vi "Monta comando comFilas .vi"(6 "Set Point":string, 7 "Comando":string, 8 "Dispositivo":string, 9 "Controlador":u16(ring)=1 items=["ZERO", "AH", "DEC", "TUBO", "CUP"]) -> (0 "Erro Comunicação":bool, 1 "String Enviado":string, 2 "Resposta":string, 3 "Erro Resp":bool)   [LabVIEW 2018]
uses:
  Global_Telescopio.vi
panel:
  out "ERRO":bool
  # "PROG"
  # "SIDERAL"
  # "EMBREAGEM"
  # "DESLIGAR"
  # "STATUS"
  # "LIGAR"
  # "PARAR"
  # "ERROS"
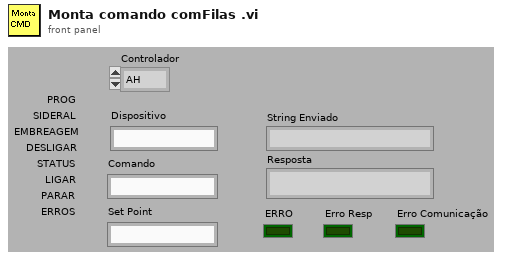
[diagram p1: front panel]
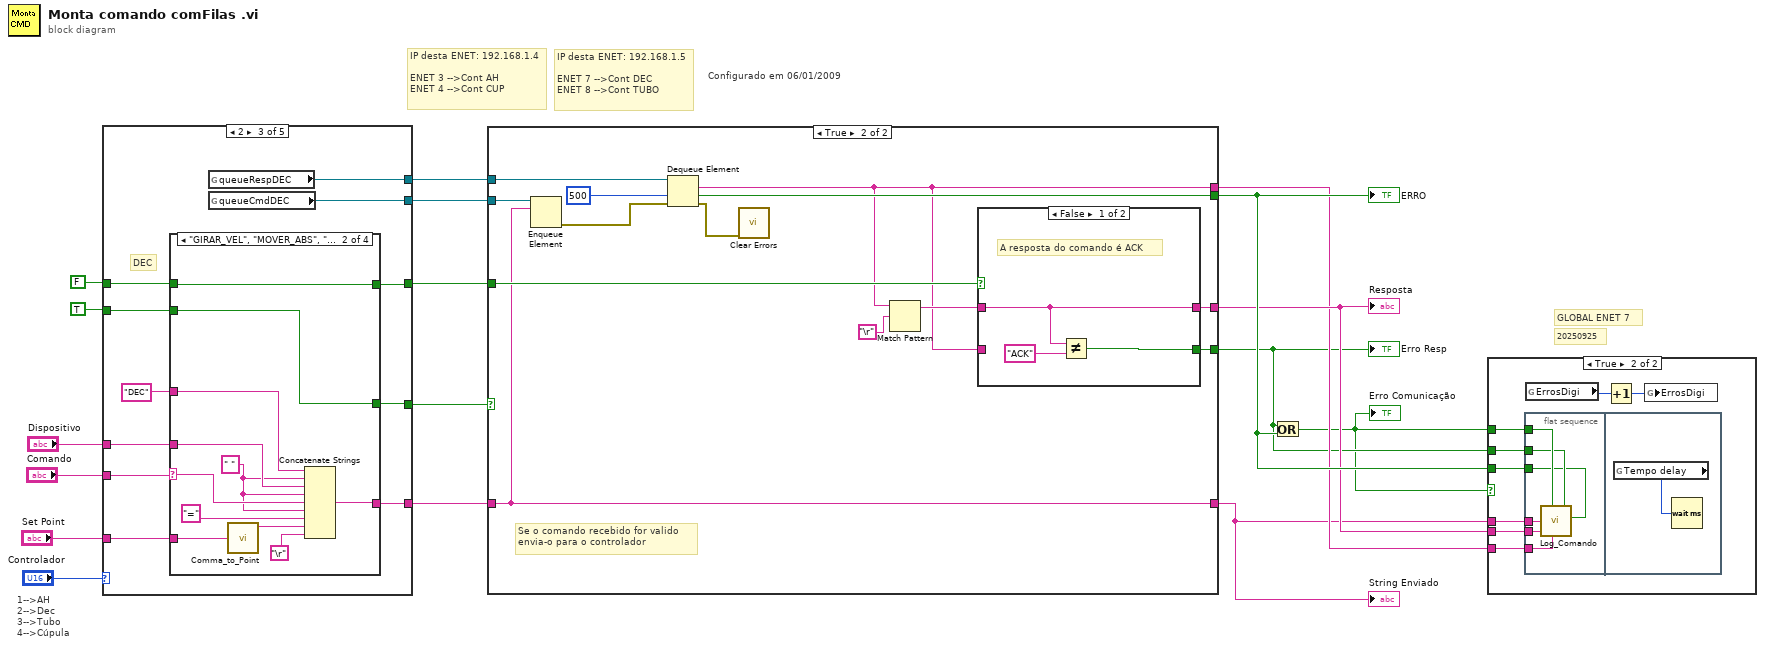
[diagram p0: block diagram]
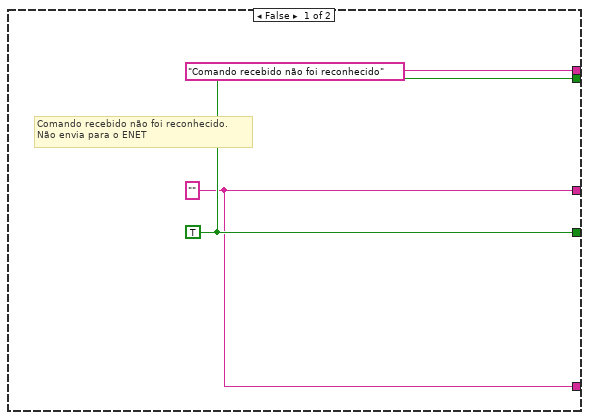
[diagram p2: hidden frame]
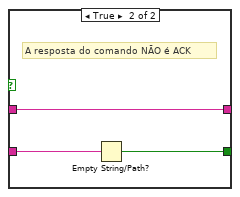
[diagram p3: hidden frame]
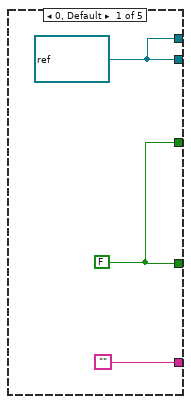
[diagram p5: hidden frame]
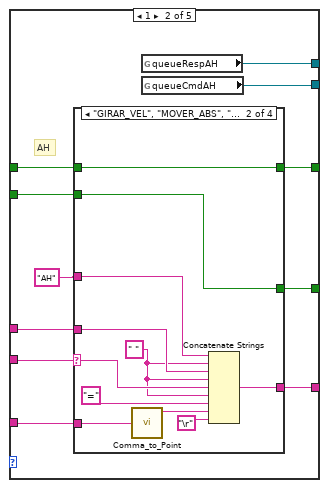
[diagram p6: hidden frame]
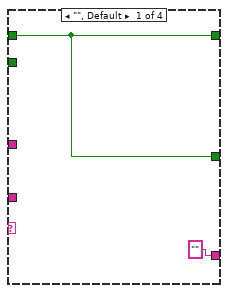
[diagram p7: hidden frame]
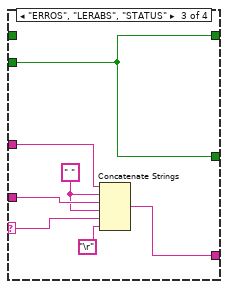
[diagram p8: hidden frame]
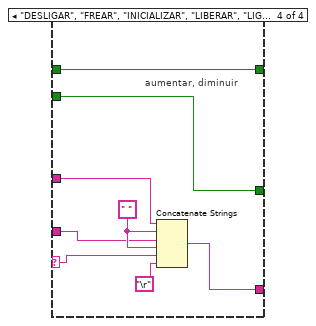
[diagram p9: hidden frame]
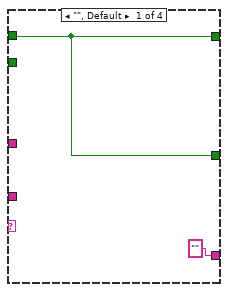
[diagram p10: hidden frame]
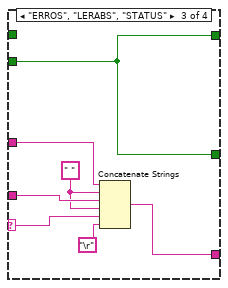
[diagram p11: hidden frame]
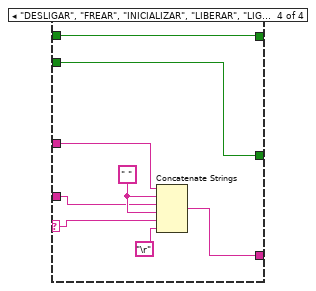
[diagram p12: hidden frame]
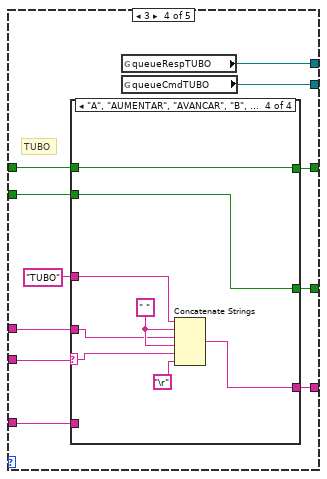
[diagram p13: hidden frame]
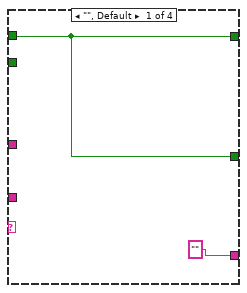
[diagram p14: hidden frame]
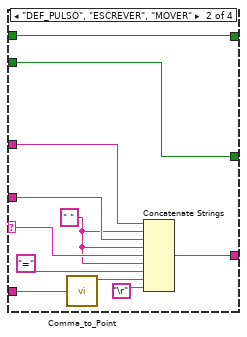
[diagram p15: hidden frame]
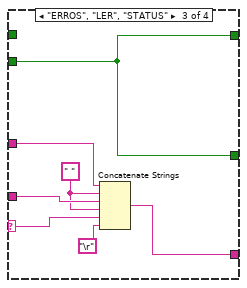
[diagram p16: hidden frame]
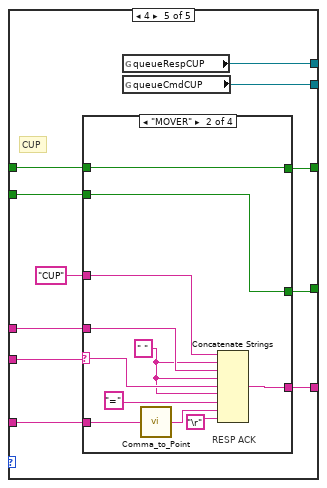
[diagram p17: hidden frame]
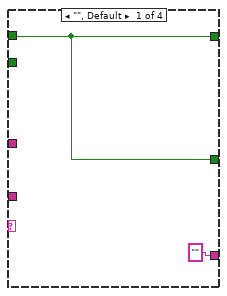
[diagram p18: hidden frame]
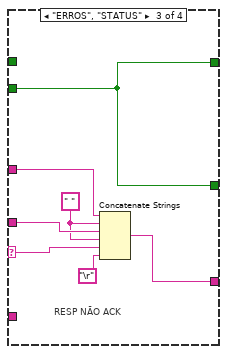
[diagram p19: hidden frame]
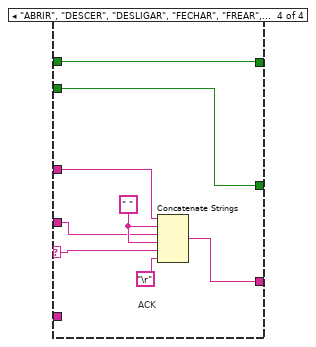
[diagram p20: hidden frame]
diagram:
  # "GLOBAL ENET 7"
  # "20250925"
  # "Configurado em 06/01/2009"
  # "IP desta ENET: 192.168.1.4\n\nENET 3 -->Cont AH\nENET 4 -->Cont CUP"
  # "IP desta ENET: 192.168.1.5\n\nENET 7 -->Cont DEC\nENET 8 -->Cont TUBO"
  # "1-->AH\n2-->Dec\n3-->Tubo\n4-->Cúpula"
  n1 = case shown="2" "Controlador" {
    tunnel: "Dispositivo" -> [_ w31 w70 w109 w148]
    tunnel: "Comando" -> [_ w30 w68 w108 w147]
    tunnel: "Set Point" -> [_ w29 w69 w107 w146]
    tunnel: ["" w28 w67 w106 w145] -> w7
    tunnel: FALSE -> [_ w27 w66 w105 w144]
    tunnel: TRUE -> [_ w26 w65 w104 w143]
    tunnel: [w20 w25 w63 w102 w141] -> w11
    tunnel: [w20 w24 w64 w103 w142] -> w10
    tunnel: [w18 w22 w61 w101 w138] -> w6
    tunnel: [w18 w23 w62 w100 w139] -> w5
    frame 0, Default {
      w18 = refnum<queue> refnum ("queueCmdCUP")
      w20 = FALSE
    }
    frame 1 {
      # "AH"
      n2 = case shown="\"GIRAR_VEL\", \"MOVER_ABS\", \"MOVER_RAP\", \"MOVER_REL\", \"SHIFT\"" w30 {
        selector: w30 -> [_ w41 w48 w54]
        tunnel: w31 -> [_ w44 w49 w55]
        tunnel: w29 -> [_ w43 _ _]
        tunnel: ["" w42 w50 w57] -> w28
        tunnel: "AH" ("string") -> [_ w40 w46 w56]
        tunnel: [w32 w39 w45 w53] -> w24
        tunnel: w27 -> [w32 w38 _ w52]
        tunnel: w26 -> [_ w39 w45 w53]
        tunnel: [w32 w38 w45 w52] -> w25
        frame "", Default {
        }
        frame "GIRAR_VEL", "MOVER_ABS", "MOVER_RAP", "MOVER_REL", "SHIFT" {
          w37 = " "
          n3 = call "Comma_to_Point.vi"("Lat_A"=w43) -> ("Saída"=w35:string)
          n4 = Concatenate Strings(w40, w37, w44, w37, w41, w37, "=", w35, "\r") -> (w42:string)
        }
        frame "ERROS", "LERABS", "STATUS" {
          w47 = " "
          n5 = Concatenate Strings(w46, w47, w49, w47, w48, "\r") -> (w50:string)
        }
        frame "DESLIGAR", "FREAR", "INICIALIZAR", "LIBERAR", "LIGAR", "PARAR", "RESET", "ZERAR" {
          w58 = " "
          # "aumentar, diminuir"
          n6 = Concatenate Strings(w56, w58, w55, w58, w54, "\r") -> (w57:string)
        }
      }
      n7 = global read "Global_Telescopio.vi" "queueRespAH"() -> (w22:refnum<queue>)
      n8 = global read "Global_Telescopio.vi" "queueCmdAH"() -> (w23:refnum<queue>)
    }
    frame 2 {
      # "DEC"
      n9 = case shown="\"GIRAR_VEL\", \"MOVER_ABS\", \"MOVER_RAP\", \"MOVER_REL\", \"SHIFT\"" w68 {
        selector: w68 -> [_ w80 w87 w93]
        tunnel: w70 -> [_ w83 w88 w94]
        tunnel: w69 -> [_ w82 _ _]
        tunnel: ["" w81 w89 w96] -> w67
        tunnel: "DEC" ("string") -> [_ w79 w85 w95]
        tunnel: [w71 w74 w84 w91] -> w64
        tunnel: w65 -> [_ w74 w84 w91]
        tunnel: w66 -> [w71 w73 _ w92]
        tunnel: [w71 w73 w84 w92] -> w63
        frame "", Default {
        }
        frame "GIRAR_VEL", "MOVER_ABS", "MOVER_RAP", "MOVER_REL", "SHIFT" {
          w78 = " "
          n10 = call "Comma_to_Point.vi"("Lat_A"=w82) -> ("Saída"=w76:string)
          n11 = Concatenate Strings(w79, w78, w83, w78, w80, w78, "=", w76, "\r") -> (w81:string)
        }
        frame "ERROS", "LERABS", "STATUS" {
          w86 = " "
          n12 = Concatenate Strings(w85, w86, w88, w86, w87, "\r") -> (w89:string)
        }
        frame "DESLIGAR", "FREAR", "INICIALIZAR", "LIBERAR", "LIGAR", "PARAR", "RESET", "ZERAR" {
          w97 = " "
          n13 = Concatenate Strings(w95, w97, w94, w97, w93, "\r") -> (w96:string)
        }
      }
      n14 = global read "Global_Telescopio.vi" "queueRespDEC"() -> (w61:refnum<queue>)
      n15 = global read "Global_Telescopio.vi" "queueCmdDEC"() -> (w62:refnum<queue>)
    }
    frame 3 {
      # "TUBO"
      n16 = case shown="\"A\", \"AUMENTAR\", \"AVANCAR\", \"B\", \"C\", \"DESLIGAR\", \"DIMINUIR\", \"GIRAR\", \"LIGAR\", \"PARAR\", \"RECUAR\", \"RESET\"" w108 {
        selector: w108 -> [_ w119 w126 w132]
        tunnel: w109 -> [_ w122 w127 w133]
        tunnel: w107 -> [_ w121 _ _]
        tunnel: ["" w120 w128 w135] -> w106
        tunnel: "TUBO" ("string") -> [_ w118 w124 w134]
        tunnel: [w110 w112 w123 w130] -> w103
        tunnel: w104 -> [_ w112 w123 w130]
        tunnel: w105 -> [w110 w113 _ w131]
        tunnel: [w110 w113 w123 w131] -> w102
        frame "", Default {
        }
        frame "DEF_PULSO", "ESCREVER", "MOVER" {
          w117 = " "
          n17 = call "Comma_to_Point.vi"("Lat_A"=w121) -> ("Saída"=w115:string)
          n18 = Concatenate Strings(w118, w117, w122, w117, w119, w117, "=", w115, "\r") -> (w120:string)
        }
        frame "ERROS", "LER", "STATUS" {
          w125 = " "
          n19 = Concatenate Strings(w124, w125, w127, w125, w126, "\r") -> (w128:string)
        }
        frame "A", "AUMENTAR", "AVANCAR", "B", "C", "DESLIGAR", "DIMINUIR", "GIRAR", "LIGAR", "PARAR", "RECUAR", "RESET" {
          w136 = " "
          n20 = Concatenate Strings(w134, w136, w133, w136, w132, "\r") -> (w135:string)
        }
      }
      n21 = global read "Global_Telescopio.vi" "queueRespTUBO"() -> (w101:refnum<queue>)
      n22 = global read "Global_Telescopio.vi" "queueCmdTUBO"() -> (w100:refnum<queue>)
    }
    frame 4 {
      # "CUP"
      n23 = case shown="\"MOVER\"" w147 {
        selector: w147 -> [_ w158 w165 w171]
        tunnel: w148 -> [_ w161 w166 w172]
        tunnel: w146 -> [_ w160 _ _]
        tunnel: ["" w159 w167 w174] -> w145
        tunnel: "CUP" ("string") -> [_ w157 w163 w173]
        tunnel: [w149 w151 w162 w169] -> w142
        tunnel: w143 -> [_ w151 w162 w169]
        tunnel: w144 -> [w149 w152 _ w170]
        tunnel: [w149 w152 w162 w170] -> w141
        frame "", Default {
        }
        frame "MOVER" {
          w156 = " "
          # "RESP ACK"
          n24 = call "Comma_to_Point.vi"("Lat_A"=w160) -> ("Saída"=w154:string)
          n25 = Concatenate Strings(w157, w156, w161, w156, w158, w156, "=", w154, "\r") -> (w159:string)
        }
        frame "ERROS", "STATUS" {
          w164 = " "
          # "RESP NÃO ACK"
          n26 = Concatenate Strings(w163, w164, w166, w164, w165, "\r") -> (w167:string)
        }
        frame "ABRIR", "DESCER", "DESLIGAR", "FECHAR", "FREAR", "GIRAR_CCW", "GIRAR_CW", "LER_LCB", "LIGAR", "LIGAR_JOG", "LIGAR_LCB", "LIGAR_RAP", "PARAR", "RESET", "SUBIR" {
          w175 = " "
          # "ACK"
          n27 = Concatenate Strings(w173, w175, w172, w175, w171, "\r") -> (w174:string)
        }
      }
      n28 = global read "Global_Telescopio.vi" "queueRespCUP"() -> (w138:refnum<queue>)
      n29 = global read "Global_Telescopio.vi" "queueCmdCUP"() -> (w139:refnum<queue>)
    }
  }
  n30 = case shown="True" w10 {
    tunnel: [w177 w191] -> w8
    tunnel: w7 -> [_ w182]
    tunnel: w11 -> [_ w192]
    tunnel: [w179 w184] -> w9
    tunnel: [w179 w190] -> w2
    tunnel: w5 -> [_ w189]
    tunnel: w6 -> [_ w186]
    tunnel: ["Comando recebido não foi reconhecido" w183] -> w4
    tunnel: [w177 w182] -> w3
    frame False {
      w179 = TRUE
      w177 = ""
      # "Comando recebido não foi reconhecido.\nNão envia para o ENET"
    }
    frame True {
      # "Se o comando recebido for valido\nenvia-o para o controlador"
      n31 = Enqueue Element(queue=w189, element=w182) -> (error out=w180:errorcluster)  [unwired: 2 in, 2 out]
      n32 = Dequeue Element(queue=w186, timeout in ms (-1)=500, error in (no error)=w180) -> (element=w183:string, timed out?=w184:bool, error out=w181:errorcluster)  [unwired: 1 out]
      n33 = call <vilib>:"Clear Errors.vi"("error in (no error)"=w181) -> ()  [unwired: 5 in, 2 out]
      n34 = Match Pattern(string=w183, regular expression="\r") -> (before substring=w187:string)  [unwired: 1 in, 3 out]
      n35 = case shown="False" w192 {
        tunnel: w187 -> [w194 w198]
        tunnel: [w194 w198] -> w191
        tunnel: [w193 w196] -> w190
        tunnel: w183 -> [_ w197]
        frame False {
          # "A resposta do comando é ACK"
          n36 = Not Equal?(x=w194, y="ACK") -> (x != y?=w193:bool)
        }
        frame True {
          # "A resposta do comando NÃO é ACK"
          n37 = Empty String/Path?(string/path=w197) -> (empty?=w196:bool)
        }
      }
    }
  }
  "Resposta" <- w8
  "String Enviado" <- w3
  "ERRO" <- w9
  "Erro Resp" <- w2
  n38 = Or(x=w2, y=w9) -> (x .or. y?=w1:bool)
  "Erro Comunicação" <- w1
  n39 = case shown="True" w1 {
    tunnel: w3 -> [_ w206]
    tunnel: w8 -> [_ w205]
    tunnel: w1 -> [_ w204]
    tunnel: w2 -> [_ w203]
    tunnel: w9 -> [_ w202]
    tunnel: w4 -> [_ w201]
    frame False {
    }
    frame True {
      n40 = flat-sequence {
        tunnel: w206 -> [w212]
        tunnel: w205 -> [w211]
        tunnel: w204 -> [w210]
        tunnel: w203 -> [w209]
        tunnel: w202 -> [w208]
        tunnel: w201 -> [w207]
        frame #0 {
          n41 = call "Log_Comando.vi"("Erro"=w210, "string do Comando"=w212, "string da resposta"=w211, "String"=w207, "Erro de Resposta"=w209, "Erro Recebido"=w208) -> ()  [unwired: 3 in]
        }
        frame #1 {
          n42 = global read "Global_Telescopio.vi" "Tempo delay"() -> (w213:i32)
          n43 = Wait (ms)(milliseconds to wait=w213) -> ()  [unwired: 1 out]
        }
      }
      n44 = global read "Global_Telescopio.vi" "ErrosDigi"() -> (w199:i16)
      n45 = Increment(x=w199) -> (x+1=w200:i16)
      n46 = global write "Global_Telescopio.vi" "ErrosDigi"(w200) -> ()
    }
  }
